vi "Get Calib Filepath.vi"(3 "Filename String":string) -> (1 "Filename Out":path)   [LabVIEW 2020]
uses:
  Globals/Meas_global.vi
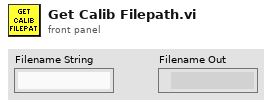
[diagram p1: front panel]
types:
  T1 = typedef "Post_Process.ctl" = enum16{"Take New Data", "Post Process Raw Data File"}
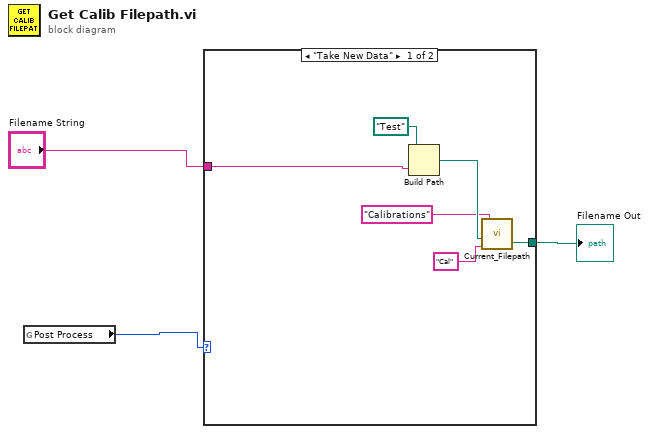
[diagram p0: block diagram]
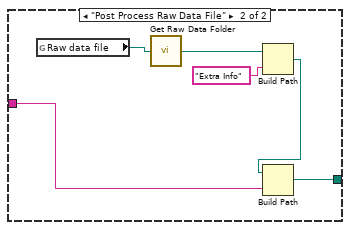
[diagram p2: hidden frame]
diagram:
  n1 = global read "Meas_global.vi" "Post Process"() -> (w2:T1)
  n2 = case shown="\"Take New Data\"" w2 {
    tunnel: [w9 w12] -> w3
    tunnel: "Filename String" -> [w7 w13]
    frame "Take New Data" {
      n3 = Build Path(base path=path "Test", name or relative path=w7) -> (appended path=w8:path)
      n4 = call "Current_Filepath.vi"("Short_Name"="Cal" ("Data Type"), "Filename in"=w8, "Data Type"="Calibrations") -> ("Filename Out"=w9:path)  [unwired: 1 in, 1 out]
    }
    frame "Post Process Raw Data File" {
      n5 = global read "Meas_global.vi" "Raw data file"() -> (w11:path)
      n6 = call "Get Raw Data Folder.vi"("Raw data file"=w11) -> ("Main Raw Data Folder"=w10:path)
      n7 = Build Path(base path=w10, name or relative path="Extra Info") -> (appended path=w14:path)
      n8 = Build Path(base path=w14, name or relative path=w13) -> (appended path=w12:path)
    }
  }
  "Filename Out" <- w3
